vi "ReadExperimentRunTimingNode.vi"(8 "Error In":errorcluster, 11 "Experiment Run Node In":refnum<k20>) -> (0 "Error Out":errorcluster, 2 "Experiment Run Timing":T1, 3 "Experiment Run Node Out":refnum<k20>)   [LabVIEW 2012]
uses:
  ExperimentRunTiming.ctl
  <vilib>/xml/NI_XML.lvlib
panel:
  out "node text 2":string
  out "node text":string
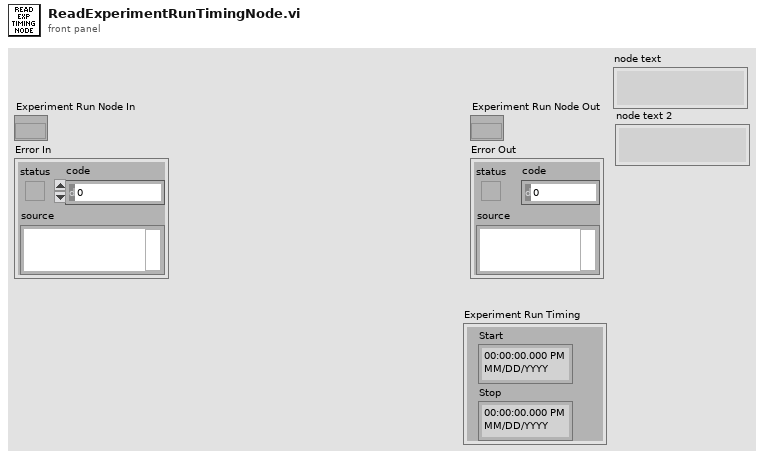
[diagram p1: front panel]
types:
  T1 = typedef "ExperimentRunTiming.ctl" = cluster{"Start":timestamp, "Stop":timestamp}
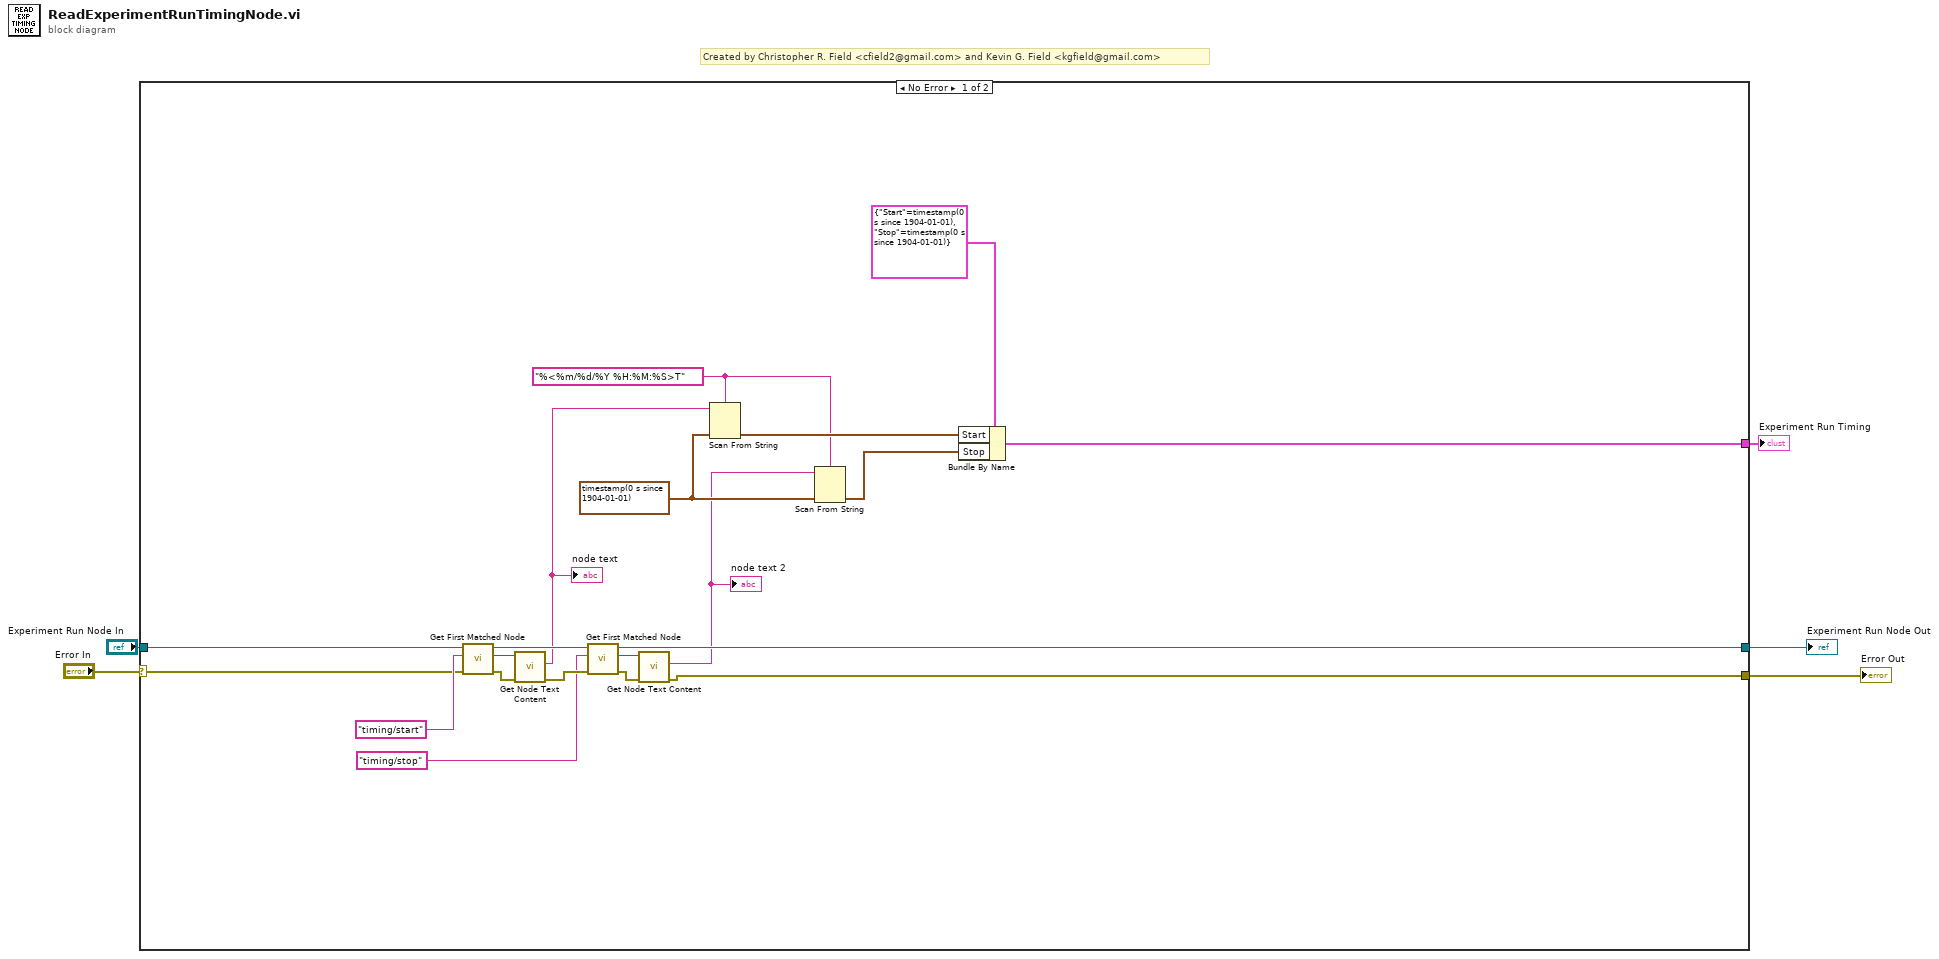
[diagram p0: block diagram]
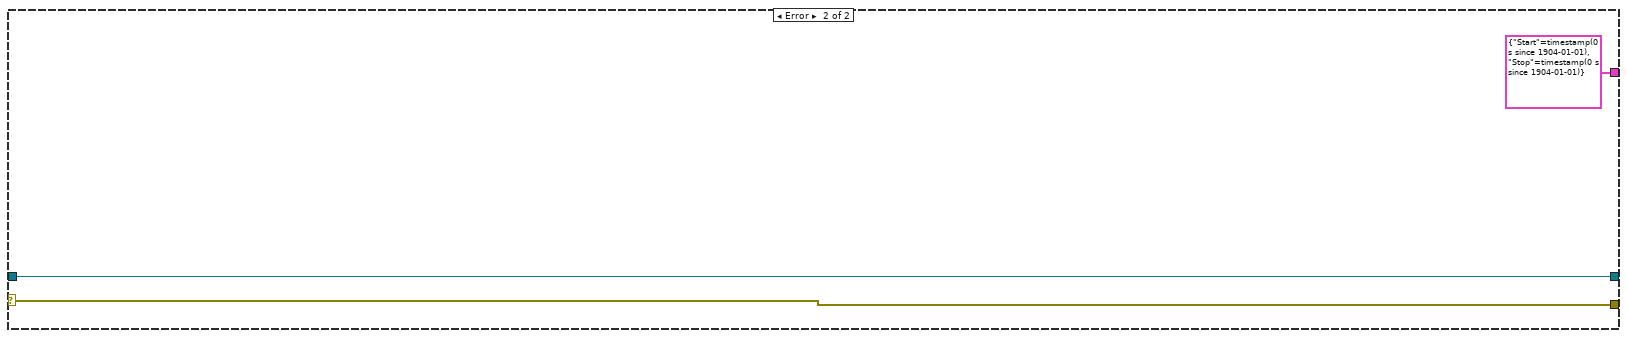
[diagram p2: hidden frame]
diagram:
  # "Created by Christopher R. Field <cfield2@gmail.com> and Kevin G. Field <kgfield@gmail.com>"
  n1 = case shown="No Error" "Error In" {
    selector: "Error In" -> [w14 w27]
    tunnel: "Experiment Run Node In" -> [w15 w28]
    tunnel: [w17 w28] -> w3
    tunnel: [w16 w27] -> w2
    tunnel: [w6 T1 {"Start"=timestamp(0 s since 1904-01-01), "Stop"=timestamp(0 s since 1904-01-01)} ("Experiment Run Timing")] -> w1
    frame No Error {
      w10 = "%<%m/%d/%Y %H:%M:%S>T" ("format string")
      w9 = timestamp(0 s since 1904-01-01)
      n2 = call <vilib>:"Get First Matched Node.vi"("error in (no error)"=w14, "XPath expression"="timing/start", "node in"=w15) -> ("error out"=w23:errorcluster, "node result"=w24:refnum<k20>, "node out"=w22:refnum<k20>)  [unwired: 6 in]
      n3 = call <vilib>:"Get Node Text Content.vi"("error in (no error)"=w23, "node in"=w24) -> ("error out"=w21:errorcluster, "node text"=w13:string)  [unwired: 7 in, 1 out]
      "node text" <- w13
      n4 = call <vilib>:"Get First Matched Node.vi"("error in (no error)"=w21, "XPath expression"="timing/stop", "node in"=w22) -> ("error out"=w18:errorcluster, "node result"=w19:refnum<k20>, "node out"=w17:refnum<k20>)  [unwired: 6 in]
      n5 = call <vilib>:"Get Node Text Content.vi"("error in (no error)"=w18, "node in"=w19) -> ("error out"=w16:errorcluster, "node text"=w8:string)  [unwired: 7 in, 1 out]
      "node text 2" <- w8
      n6 = Scan From String(format string=w10, input string=w13, default 1=w9) -> (output 1=w11:timestamp)  [unwired: 2 in, 3 out]
      n7 = Scan From String(format string=w10, input string=w8, default 1=w9) -> (output 1=w7:timestamp)  [unwired: 2 in, 3 out]
      n8 = Bundle By Name(cluster=T1 {"Start"=timestamp(0 s since 1904-01-01), "Stop"=timestamp(0 s since 1904-01-01)} ("Experiment Run Timing"), "Start"=w11, "Stop"=w7) -> (w6:T1)
    }
    frame Error {
    }
  }
  "Experiment Run Node Out" <- w3
  "Error Out" <- w2
  "Experiment Run Timing" <- w1
